vi "Insight_Telnet_VI_Test.vi"() -> ()   [LabVIEW 2011]
uses:
  Telnet Session.ctl
panel:
  out "Index of Synch Pulse":u32
  in  "Laser Write Values":T1={"Clock Rate (MHz)"=400.0, "num points"=0, "Duty Cycle (%)"=50.0, "Repetition Rate (kHz)"=200.0, "Start Wavelength (nm)"=1520.0, "Stop Wavelength (nm)"=1570.0, "Power (mW)"=1.0, "Power Profile"=enum."FLAT", "Sample Clock Delay (nsec)"=0.0, "Sweep Start Delay (nsec)"=0.0, "Data Valid Delay (nsec)"=0.0, "Optical Freq. Step (GHz)"=0.0, "Data Vector Length"=2000, "OPC Bit"=0}
  out "Invalid Data Indices":i32[](array[numeric])
  out "PLev Execution Timer (s)":dbl
  out "*IDN?":string
  out "Read Laser Settings":T1={"Clock Rate (MHz)"=400.0, "num points"=0, "Duty Cycle (%)"=50.0, "Repetition Rate (kHz)"=200.0, "Start Wavelength (nm)"=1520.0, "Stop Wavelength (nm)"=1570.0, "Power (mW)"=1.0, "Power Profile"=enum."FLAT", "Sample Clock Delay (nsec)"=0.0, "Sweep Start Delay (nsec)"=0.0, "Data Valid Delay (nsec)"=0.0, "Optical Freq. Step (GHz)"=0.0, "Data Vector Length"=2000, "OPC Bit"=0}
  in  "Mode":enum8{"Write", "Read"}(ring)=enum."Read"
  in  "Laser CMDs":T2(ring)
  in  "stop":bool
  out "error out":errorcluster
  in  "error in (no error)":errorcluster
  in  "IP Address":string="192.168.0.222"
  in  "Send Command":bool
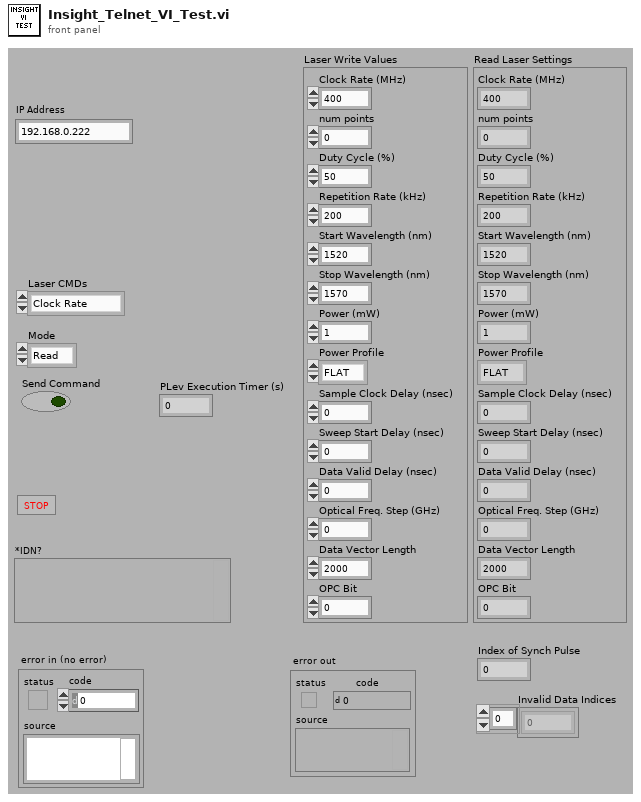
[diagram p1: front panel]
types:
  T1 = cluster{"Clock Rate (MHz)":dbl, "num points":u32, "Duty Cycle (%)":dbl, "Repetition Rate (kHz)":dbl, "Start Wavelength (nm)":dbl, "Stop Wavelength (nm)":dbl, "Power (mW)":dbl, "Power Profile":enum16{"FLAT", "GAUSsian"}, "Sample Clock Delay (nsec)":dbl, "Sweep Start Delay (nsec)":dbl, "Data Valid Delay (nsec)":dbl, "Optical Freq. Step (GHz)":dbl, "Data Vector Length":i32, "OPC Bit":u32}
  T2 = enum16{"Clock Rate", "Num Points", "Total Points", "Rep Rate", "DVV", "Freq Step", "StartWL", "StopWL", "Power", "Profile", "SCDelay", "SSDelay", "DVDelay", "Sync Index", "Synch Pulse", "Calibrate", "Abort", "Check OPC", "Get Parameters", "Power-Level", "Init Sweep"}
  T3 = typedef "Telnet Session.ctl" = refnum<k1>
  T4 = cluster{"Save Data Path":path, "Laser Serial Port":refnum<visa-resource-name>, "IP address":string, "remote port or service name":u16, "Laser connection ID":refnum<k5>, "telnet connection":T3, "*IDN":string, "OPC Bit":u32, "Counter":u32, "Measurement Complete?":bool, "Speed of Light (GHz-mm)":dbl, "Laser State":enum16{"Standby", "Calibrate", "Scan", "Fixed", "Idle"}, "Clock Rate (MHz)":dbl, "DAC Repeats":u32, "num points":u32, "Duty Cycle (%)":dbl, "Repetition Rate (kHz)":dbl, "Start Wavelength (nm)":dbl, "Stop Wavelength (nm)":dbl, "Power (mW)":dbl, "Power Profile":enum16{"FLAT", "GAUSsian"}, "Sample Clock Delay (nsec)":dbl, "Sweep Start Delay (nsec)":dbl, "Data Valid Delay (nsec)":dbl, "FFT Window":enum16{"Rectangular", "Hanning", "Hamming", "Blackman", "Blackman-Harris"}, "Data Vector Length":u32, "Optical Freq. Step (GHz)":dbl, "Distance Step (um)":dbl, "Indices of Data Invalid":i32[], "Raw Data":dbl[], "Data Valid":dbl[], "Processed Data":dbl[], "PSF":dbl[], "Distance Axis (mm)":dbl[], "Number of Measurements":i32, "PSF DataOut":cluster{"FW@3dB":dbl, "FW@20dB":dbl, "Ypeak":dbl, "Xpeak":dbl, "Dynamic \nRange":dbl, "WLRange (nm)":dbl}, "Program Message":string, "Data Acquisition Card":enum16{"Alazar Tech ATS9350", "SP Devices ADQ214"}, "adq_cu_ptr":u32, "adq214_num":i32, "Actual Laser Settings":cluster{"Clock Rate (MHz)":dbl, "num points":u32, "Duty Cycle (%)":dbl, "Repetition Rate (kHz)":dbl, "Start Wavelength (nm)":dbl, "Stop Wavelength (nm)":dbl, "Power (mW)":dbl, "Power Profile":enum16{"FLAT", "GAUSsian"}, "Sample Clock Delay (nsec)":dbl, "Sweep Start Delay (nsec)":dbl, "Data Valid Delay (nsec)":dbl, "Optical Freq. Step (GHz)":dbl, "Data Vector Length":i32, "OPC Bit":u32}, "Synch Data":dbl[][]}
  T5 = enum16{"Standby", "Calibrate", "Scan", "Fixed", "Idle"}
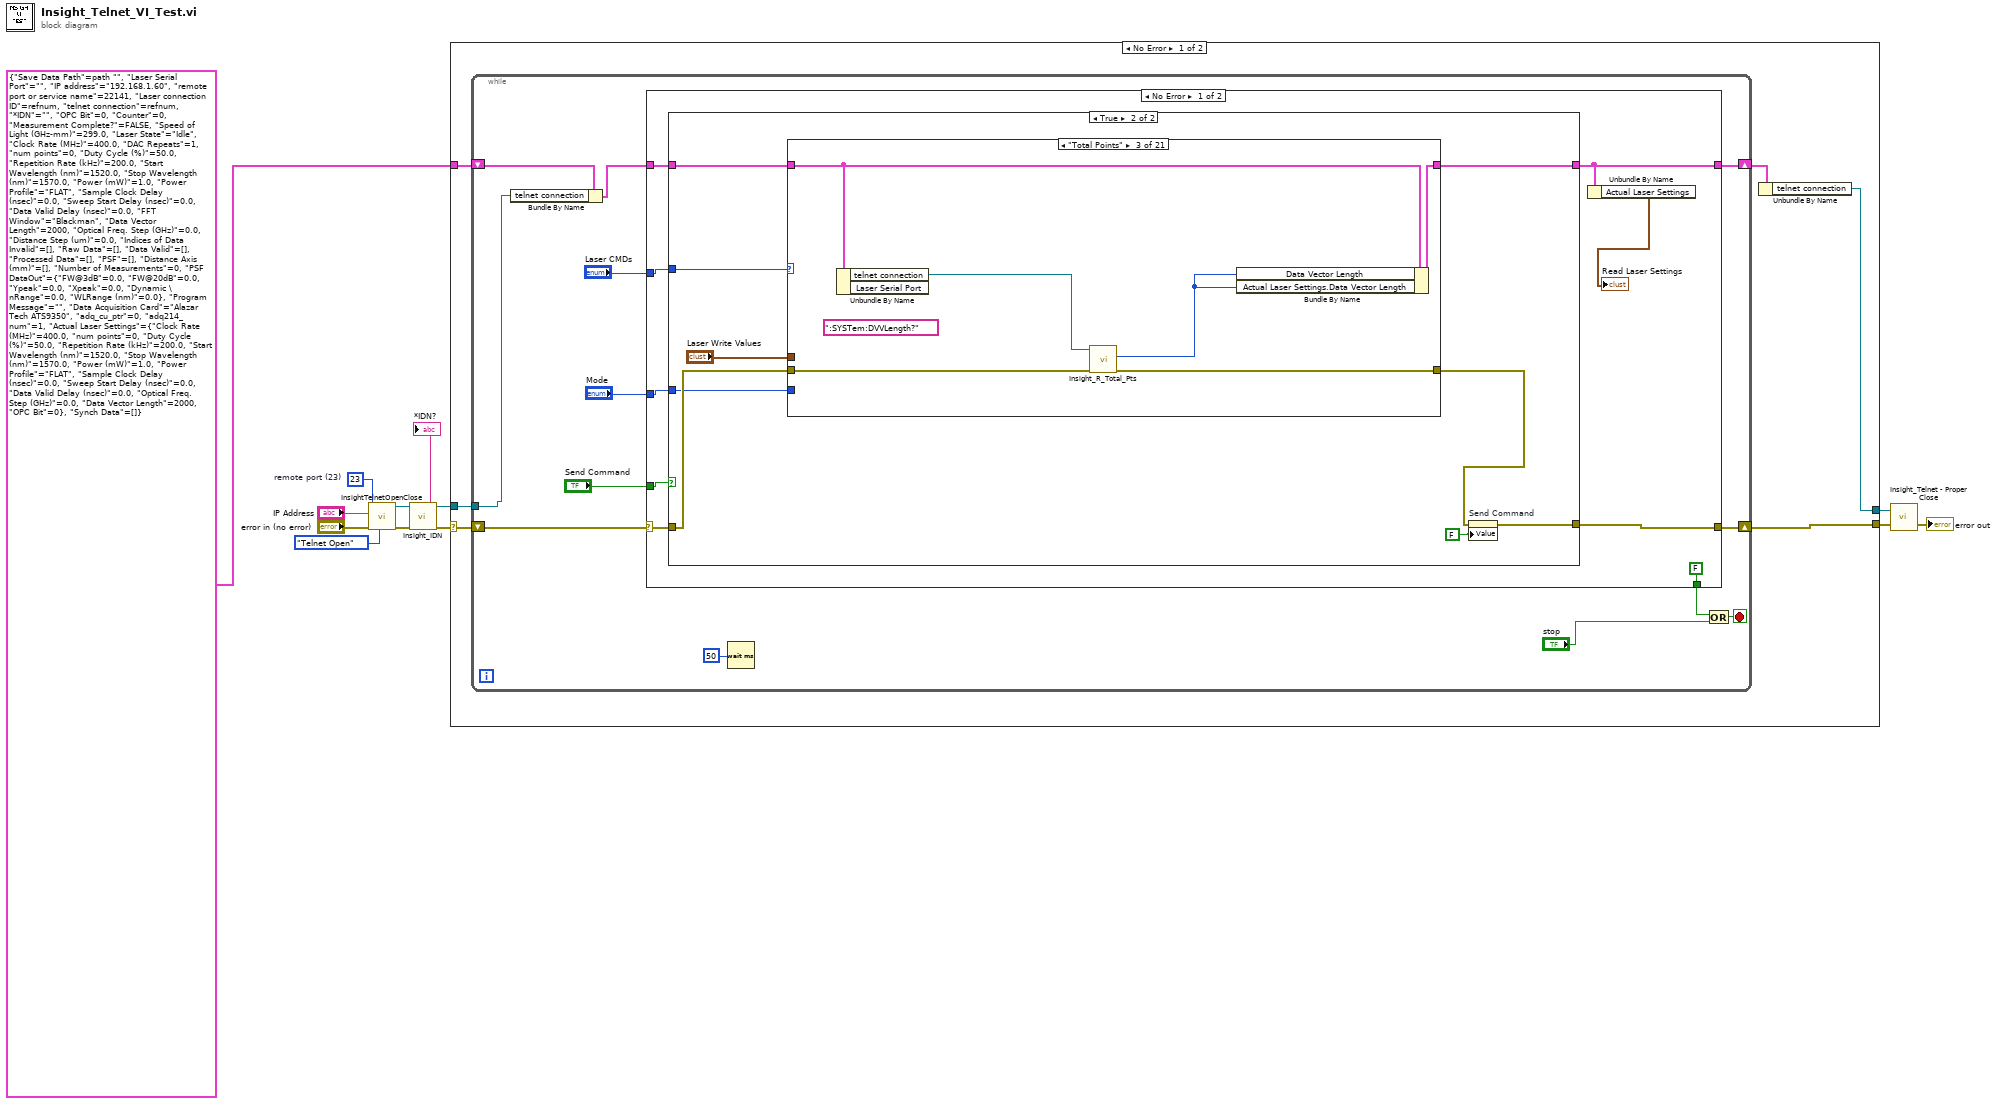
[diagram p0: block diagram]
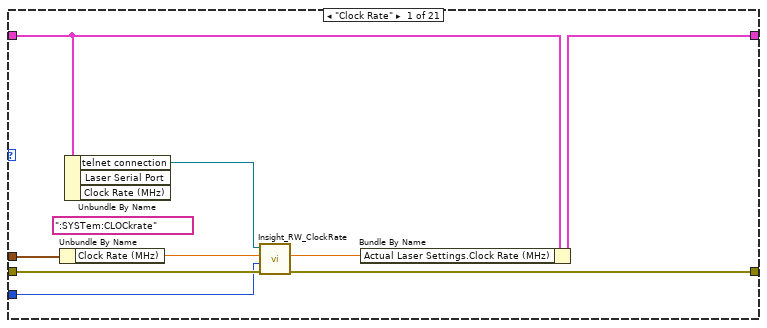
[diagram p3: hidden frame]
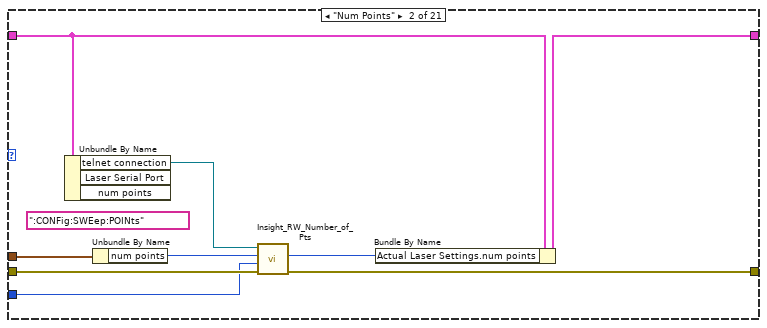
[diagram p4: hidden frame]
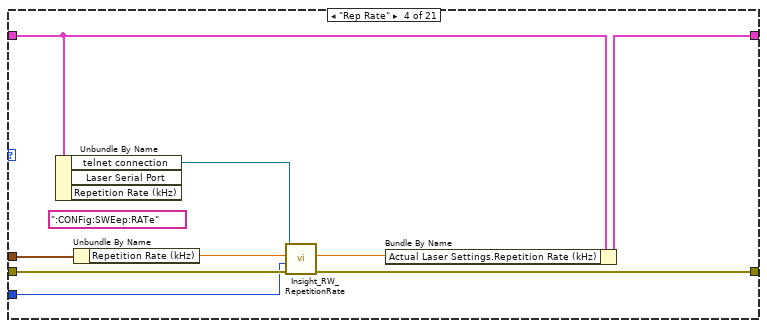
[diagram p5: hidden frame]
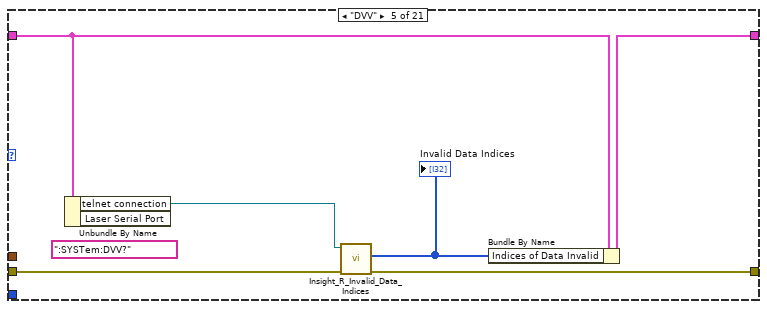
[diagram p6: hidden frame]
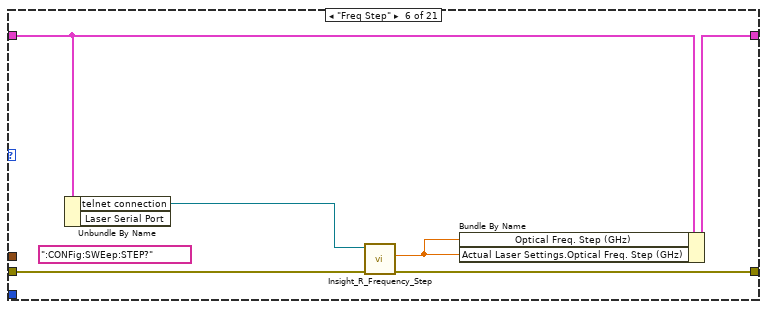
[diagram p7: hidden frame]
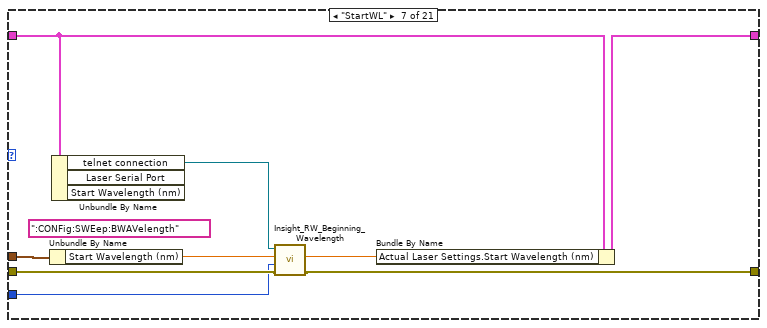
[diagram p8: hidden frame]
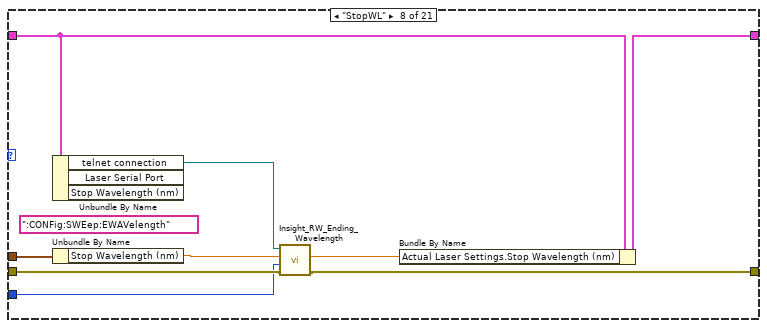
[diagram p9: hidden frame]
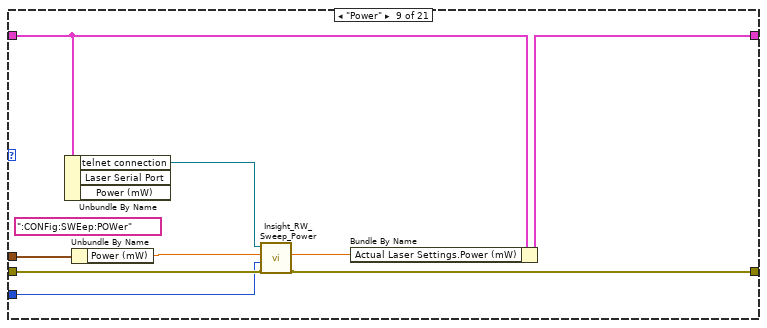
[diagram p10: hidden frame]
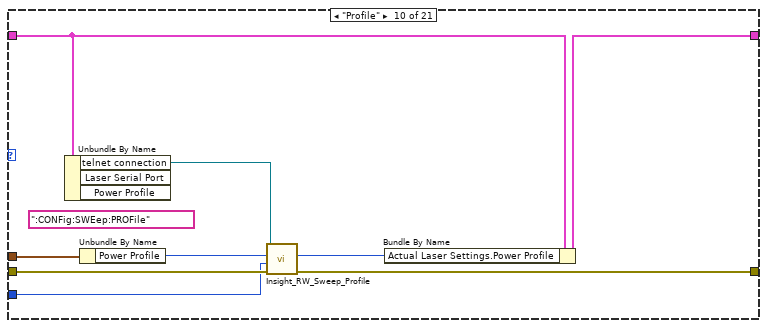
[diagram p11: hidden frame]
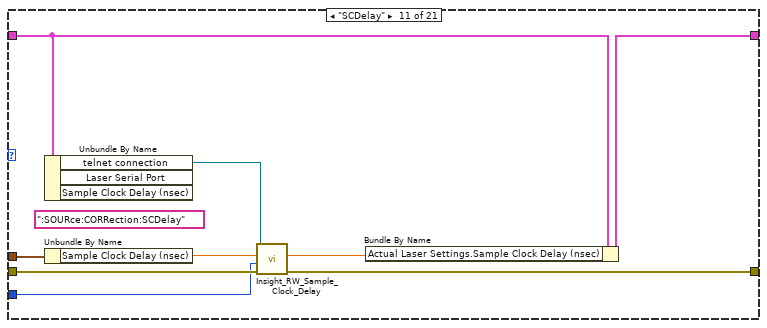
[diagram p12: hidden frame]
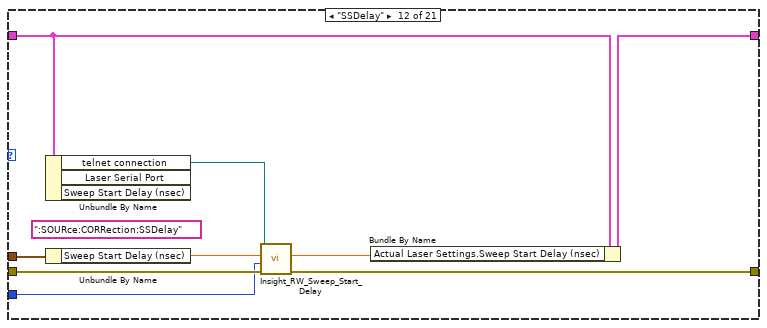
[diagram p13: hidden frame]
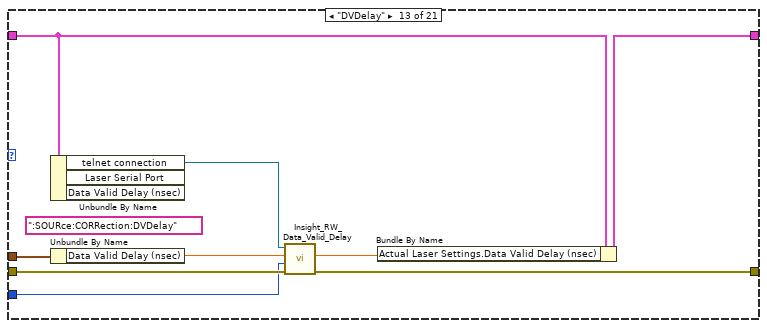
[diagram p14: hidden frame]
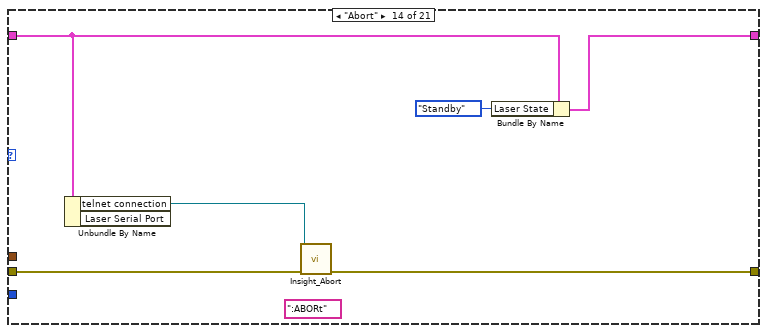
[diagram p15: hidden frame]
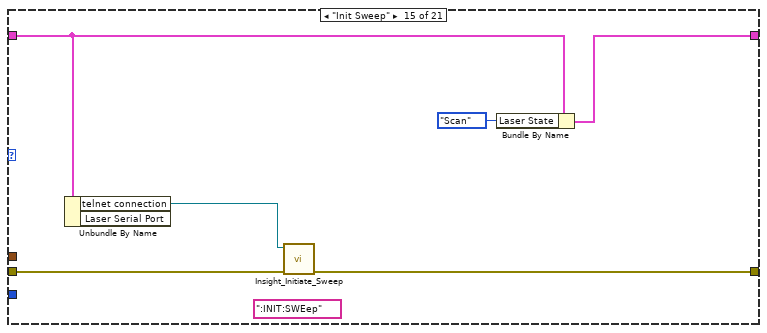
[diagram p16: hidden frame]
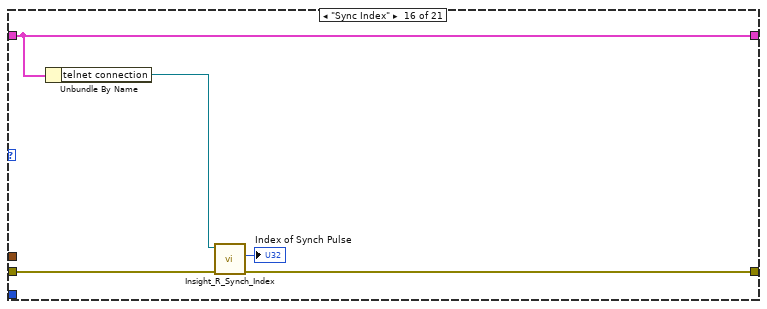
[diagram p17: hidden frame]
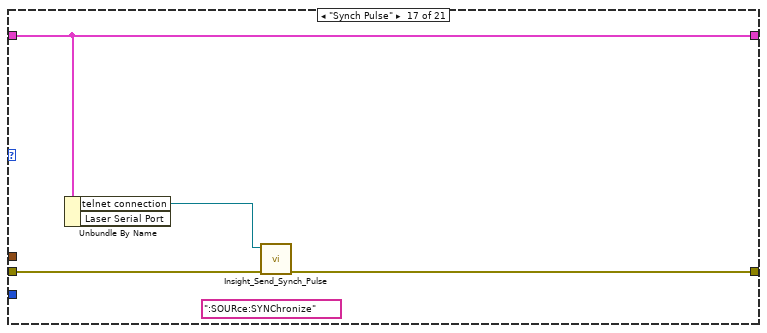
[diagram p18: hidden frame]
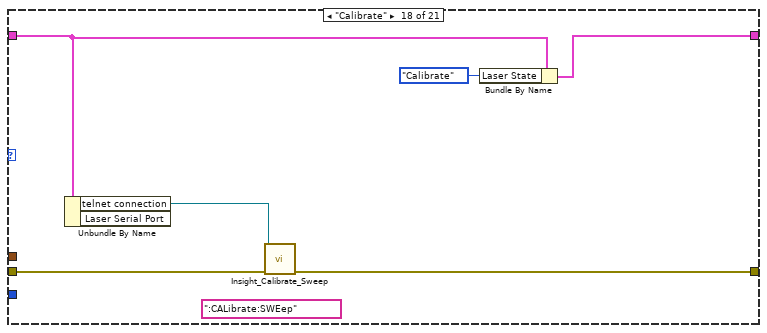
[diagram p19: hidden frame]
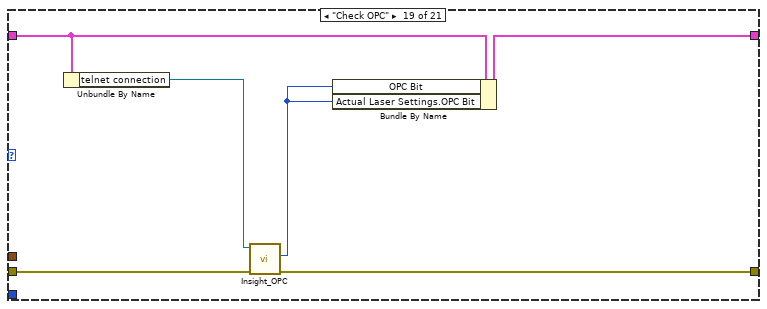
[diagram p20: hidden frame]
diagram:
  w1 = u16 23  # remote port (23)
  n1 = call "InsightTelnetOpenClose.vi"("IP Address"="IP Address", "remote port (23)"=w1, "error in (no error)"="error in (no error)", "Method"=enum16{"Telnet Open", "Telnet Close"}."Telnet Open") -> ("telnet connection"=w4:T3, "error out"=w6:errorcluster)  [unwired: 5 in]
  n2 = call "Insight_IDN.vi"("error in (no error)"=w6, "telnet connection"=w4) -> ("error out"=w5:errorcluster, "*IDN?"=→"*IDN?":string, "telnet  connection out"=w3:T3)  [unwired: 7 in]
  n3 = case shown="No Error" w5 {
    selector: w5 -> [w17 w220]
    tunnel: [w18 w220] -> w13
    tunnel: w3 -> [w19 w219]
    tunnel: [w14 w219] -> w12
    tunnel: T4 {"Save Data Path"=path "", "Laser Serial Port"="", "IP address"="192.168.1.60", "remote port or service name"=22141, "Laser connection ID"=refnum, "telnet connection"=refnum, "*IDN"="", "OPC Bit"=0, "Counter"=0, "Measurement Complete?"=FALSE, "Speed of Light (GHz-mm)"=299.0, "Laser State"=enum."Idle", "Clock Rate (MHz)"=400.0, "DAC Repeats"=1, "num points"=0, "Duty Cycle (%)"=50.0, "Repetition Rate (kHz)"=200.0, "Start Wavelength (nm)"=1520.0, "Stop Wavelength (nm)"=1570.0, "Power (mW)"=1.0, "Power Profile"=enum."FLAT", "Sample Clock Delay (nsec)"=0.0, "Sweep Start Delay (nsec)"=0.0, "Data Valid Delay (nsec)"=0.0, "FFT Window"=enum."Blackman", "Data Vector Length"=2000, "Optical Freq. Step (GHz)"=0.0, "Distance Step (um)"=0.0, "Indices of Data Invalid"=[], "Raw Data"=[], "Data Valid"=[], "Processed Data"=[], "PSF"=[], "Distance Axis (mm)"=[], "Number of Measurements"=0, "PSF DataOut"={"FW@3dB"=0.0, "FW@20dB"=0.0, "Ypeak"=0.0, "Xpeak"=0.0, "Dynamic \nRange"=0.0, "WLRange (nm)"=0.0}, "Program Message"="", "Data Acquisition Card"=enum."Alazar Tech ATS9350", "adq_cu_ptr"=0, "adq214_num"=1, "Actual Laser Settings"={"Clock Rate (MHz)"=400.0, "num points"=0, "Duty Cycle (%)"=50.0, "Repetition Rate (kHz)"=200.0, "Start Wavelength (nm)"=1520.0, "Stop Wavelength (nm)"=1570.0, "Power (mW)"=1.0, "Power Profile"=enum."FLAT", "Sample Clock Delay (nsec)"=0.0, "Sweep Start Delay (nsec)"=0.0, "Data Valid Delay (nsec)"=0.0, "Optical Freq. Step (GHz)"=0.0, "Data Vector Length"=2000, "OPC Bit"=0}, "Synch Data"=[]} -> [w16 _]
    frame No Error {
      n4 = while {
        tunnel: w19 -> [w20]
        shift-right: [w30] -> w18
        shift-left: w17 -> [w29]
        shift-right: [w25] -> w15
        shift-left: w16 -> [w22]
        stop <- w26 stop-if-true
        n5 = Bundle By Name(cluster=w22, "telnet connection"=w20) -> (w21:T4)
        n6 = case shown="No Error" w29 {
          selector: w29 -> [w39 w218]
          tunnel: "Send Command" -> [w41 _]
          tunnel: [w40 w218] -> w30
          tunnel: [FALSE TRUE] -> w28
          tunnel: w21 -> [w37 w216]
          tunnel: [w34 w216] -> w25
          tunnel: "Laser CMDs" -> [w36 _]
          tunnel: "Mode" -> [w35 _]
          frame No Error {
            n7 = case shown="True" w41 {
              tunnel: w39 -> [w43 w47]
              tunnel: [w43 w51] -> w40
              tunnel: w37 -> [w42 w49]
              tunnel: [w42 w48] -> w34
              tunnel: w36 -> [_ w46]
              tunnel: w35 -> [_ w45]
              frame False {
              }
              frame True {
                n8 = case shown="\"Total Points\"" w46 {
                  tunnel: w49 -> [w61 w70 w76 w85 w91 w97 w106 w115 w124 w133 w142 w151 w160 w166 w172 w177 w181 w186 w190 w195 w197]
                  tunnel: w47 -> [w59 w68 w74 w83 w89 w95 w104 w113 w122 w131 w140 w149 w158 w162 w169 w176 w179 w184 w193 w194 w203]
                  tunnel: [w60 w69 w75 w84 w90 w96 w105 w114 w123 w132 w141 w150 w159 w165 w171 w177 w181 w185 w189 w195 w197] -> w48
                  tunnel: [w58 w67 w73 w82 w88 w94 w103 w112 w121 w130 w139 w148 w157 w161 w168 w174 w180 w183 w192 w194 w198] -> w50
                  tunnel: w45 -> [w55 w64 _ w79 _ _ w101 w110 w118 w129 w136 w145 w154 _ _ _ _ _ _ _ _]
                  tunnel: "Laser Write Values" -> [w54 w63 _ w77 _ _ w99 w108 w117 w126 w135 w144 w153 _ _ _ _ _ _ _ _]
                  frame "Clock Rate" {
                    (unwired) ":SYSTem:CLOCkrate" ("String")
                    n9 = Unbundle By Name(w54) -> ("Clock Rate (MHz)"=w53:dbl)
                    n10 = Unbundle By Name(w61) -> ("telnet connection"=w56:T3)  [unwired: 2 out]
                    n11 = call "Insight_RW_ClockRate.vi"("error in (no error)"=w59, "Mode (Read / Write)"=w55, "Clock Rate (MHz)"=w53, "telnet connection"=w56) -> ("error out"=w58:errorcluster, "Clock Rate (MHz)"=w57:dbl)  [unwired: 4 in, 2 out]
                    n12 = Bundle By Name(cluster=w61, "Actual Laser Settings.Clock Rate (MHz)"=w57) -> (w60:T4)
                  }
                  frame "Num Points" {
                    (unwired) ":CONFig:SWEep:POINts" ("String")
                    n13 = Unbundle By Name(w70) -> ("telnet connection"=w65:T3)  [unwired: 2 out]
                    n14 = Unbundle By Name(w63) -> ("num points"=w62:u32)
                    n15 = call "Insight_RW_Number_of_Pts.vi"("error in (no error)"=w68, "Mode (Read / Write)"=w64, "Number of Points"=w62, "telnet connection"=w65) -> ("error out"=w67:errorcluster, "Number of Points"=w66:u32)  [unwired: 4 in, 2 out]
                    n16 = Bundle By Name(cluster=w70, "Actual Laser Settings.num points"=w66) -> (w69:T4)
                  }
                  frame "Total Points" {
                    (unwired) ":SYSTem:DVVLength?" ("String")
                    n17 = Unbundle By Name(w76) -> ("telnet connection"=w71:T3)  [unwired: 1 out]
                    n18 = call "Insight_R_Total_Pts.vi"("error in (no error)"=w74, "telnet connection"=w71) -> ("error out"=w73:errorcluster, "Total Points"=w72:u32)  [unwired: 6 in, 2 out]
                    n19 = Bundle By Name(cluster=w76, "Data Vector Length"=w72, "Actual Laser Settings.Data Vector Length"=w72) -> (w75:T4)
                  }
                  frame "Rep Rate" {
                    (unwired) ":CONFig:SWEep:RATe" ("String")
                    n20 = Unbundle By Name(w85) -> ("telnet connection"=w80:T3)  [unwired: 2 out]
                    n21 = Unbundle By Name(w77) -> ("Repetition Rate (kHz)"=w78:dbl)
                    n22 = call "Insight_RW_RepetitionRate.vi"("error in (no error)"=w83, "Mode (Read / Write)"=w79, "Repetition Rate (kHz)"=w78, "telnet connection"=w80) -> ("error out"=w82:errorcluster, "Repetition Rate (kHz)"=w81:dbl)  [unwired: 4 in, 2 out]
                    n23 = Bundle By Name(cluster=w85, "Actual Laser Settings.Repetition Rate (kHz)"=w81) -> (w84:T4)
                  }
                  frame "DVV" {
                    (unwired) ":SYSTem:DVV?" ("String")
                    n24 = Unbundle By Name(w91) -> ("telnet connection"=w87:T3)  [unwired: 1 out]
                    n25 = call "Insight_R_Invalid_Data_Indices.vi"("error in (no error)"=w89, "telnet connection"=w87) -> ("error out"=w88:errorcluster, "Invalid Data Indices"=w86:i32[])  [unwired: 6 in, 2 out]
                    "Invalid Data Indices" <- w86
                    n26 = Bundle By Name(cluster=w91, "Indices of Data Invalid"=w86) -> (w90:T4)
                  }
                  frame "Freq Step" {
                    (unwired) ":CONFig:SWEep:STEP?" ("String")
                    n27 = Unbundle By Name(w97) -> ("telnet connection"=w93:T3)  [unwired: 1 out]
                    n28 = call "Insight_R_Frequency_Step.vi"("error in (no error)"=w95, "telnet connection"=w93) -> ("error out"=w94:errorcluster, "Optical Frequency Step (GHz)"=w92:dbl)  [unwired: 6 in, 2 out]
                    n29 = Bundle By Name(cluster=w97, "Optical Freq. Step (GHz)"=w92, "Actual Laser Settings.Optical Freq. Step (GHz)"=w92) -> (w96:T4)
                  }
                  frame "StartWL" {
                    (unwired) ":CONFig:SWEep:BWAVelength" ("String")
                    n30 = Unbundle By Name(w99) -> ("Start Wavelength (nm)"=w98:dbl)
                    n31 = Unbundle By Name(w106) -> ("telnet connection"=w102:T3)  [unwired: 2 out]
                    n32 = call "Insight_RW_Beginning_Wavelength.vi"("error in (no error)"=w104, "Mode (Read / Write)"=w101, "Beginning Wavelength (nm)"=w98, "telnet connection"=w102) -> ("error out"=w103:errorcluster, "Beginning Wavelength (nm)"=w100:dbl)  [unwired: 4 in, 2 out]
                    n33 = Bundle By Name(cluster=w106, "Actual Laser Settings.Start Wavelength (nm)"=w100) -> (w105:T4)
                  }
                  frame "StopWL" {
                    (unwired) ":CONFig:SWEep:EWAVelength" ("String")
                    n34 = Unbundle By Name(w115) -> ("telnet connection"=w111:T3)  [unwired: 2 out]
                    n35 = Unbundle By Name(w108) -> ("Stop Wavelength (nm)"=w107:dbl)
                    n36 = call "Insight_RW_Ending_Wavelength.vi"("error in (no error)"=w113, "Mode (Read / Write)"=w110, "Ending Wavelength (nm)"=w107, "telnet connection"=w111) -> ("error out"=w112:errorcluster, "Ending Wavelength (nm)"=w109:dbl)  [unwired: 4 in, 2 out]
                    n37 = Bundle By Name(cluster=w115, "Actual Laser Settings.Stop Wavelength (nm)"=w109) -> (w114:T4)
                  }
                  frame "Power" {
                    (unwired) ":CONFig:SWEep:POWer" ("String")
                    n38 = Unbundle By Name(w124) -> ("telnet connection"=w119:T3)  [unwired: 2 out]
                    n39 = Unbundle By Name(w117) -> ("Power (mW)"=w116:dbl)
                    n40 = call "Insight_RW_Sweep_Power.vi"("error in (no error)"=w122, "Mode (Read / Write)"=w118, "Power (mW)"=w116, "telnet connection"=w119) -> ("error out"=w121:errorcluster, "Power (mW)"=w120:dbl)  [unwired: 4 in, 2 out]
                    n41 = Bundle By Name(cluster=w124, "Actual Laser Settings.Power (mW)"=w120) -> (w123:T4)
                  }
                  frame "Profile" {
                    (unwired) ":CONFig:SWEep:PROFile" ("String")
                    n42 = Unbundle By Name(w133) -> ("telnet connection"=w128:T3)  [unwired: 2 out]
                    n43 = Unbundle By Name(w126) -> ("Power Profile"=w125:enum16{"FLAT", "GAUSsian"})
                    n44 = call "Insight_RW_Sweep_Profile.vi"("error in (no error)"=w131, "Mode (Read / Write)"=w129, "Power Profile"=w125, "telnet connection"=w128) -> ("error out"=w130:errorcluster, "Power Profile"=w127:enum16{"FLAT", "GAUSsian"})  [unwired: 4 in, 2 out]
                    n45 = Bundle By Name(cluster=w133, "Actual Laser Settings.Power Profile"=w127) -> (w132:T4)
                  }
                  frame "SCDelay" {
                    (unwired) ":SOURce:CORRection:SCDelay" ("String")
                    n46 = Unbundle By Name(w142) -> ("telnet connection"=w138:T3)  [unwired: 2 out]
                    n47 = Unbundle By Name(w135) -> ("Sample Clock Delay (nsec)"=w134:dbl)
                    n48 = call "Insight_RW_Sample_Clock_Delay.vi"("error in (no error)"=w140, "Mode (Read / Write)"=w136, "Sample Clock Delay (nsec)"=w134, "telnet connection"=w138) -> ("error out"=w139:errorcluster, "Sample Clock Delay (nsec)"=w137:dbl)  [unwired: 4 in, 2 out]
                    n49 = Bundle By Name(cluster=w142, "Actual Laser Settings.Sample Clock Delay (nsec)"=w137) -> (w141:T4)
                  }
                  frame "SSDelay" {
                    (unwired) ":SOURce:CORRection:SSDelay" ("String")
                    n50 = Unbundle By Name(w151) -> ("telnet connection"=w146:T3)  [unwired: 2 out]
                    n51 = Unbundle By Name(w144) -> ("Sweep Start Delay (nsec)"=w143:dbl)
                    n52 = call "Insight_RW_Sweep_Start_Delay.vi"("error in (no error)"=w149, "Mode (Read / Write)"=w145, "Sweep Start Delay (nsec)"=w143, "telnet connection"=w146) -> ("error out"=w148:errorcluster, "Sweep Start Delay (nsec)"=w147:dbl)  [unwired: 4 in, 2 out]
                    n53 = Bundle By Name(cluster=w151, "Actual Laser Settings.Sweep Start Delay (nsec)"=w147) -> (w150:T4)
                  }
                  frame "DVDelay" {
                    (unwired) ":SOURce:CORRection:DVDelay" ("String")
                    n54 = Unbundle By Name(w160) -> ("telnet connection"=w155:T3)  [unwired: 2 out]
                    n55 = Unbundle By Name(w153) -> ("Data Valid Delay (nsec)"=w152:dbl)
                    n56 = call "Insight_RW_Data_Valid_Delay.vi"("error in (no error)"=w158, "Mode (Read / Write)"=w154, "Data Valid Delay (nsec)"=w152, "telnet connection"=w155) -> ("error out"=w157:errorcluster, "Data Valid Delay (nsec)"=w156:dbl)  [unwired: 4 in, 2 out]
                    n57 = Bundle By Name(cluster=w160, "Actual Laser Settings.Data Valid Delay (nsec)"=w156) -> (w159:T4)
                  }
                  frame "Abort" {
                    (unwired) ":ABORt" ("String")
                    n58 = Unbundle By Name(w166) -> ("telnet connection"=w163:T3)  [unwired: 1 out]
                    n59 = call "Insight_Abort.vi"("error in (no error)"=w162, "telnet connection"=w163) -> ("error out"=w161:errorcluster)  [unwired: 7 in, 2 out]
                    n60 = Bundle By Name(cluster=w166, "Laser State"=T5."Standby") -> (w165:T4)
                  }
                  frame "Init Sweep" {
                    (unwired) ":INIT:SWEep" ("String")
                    n61 = Unbundle By Name(w172) -> ("telnet connection"=w167:T3)  [unwired: 1 out]
                    n62 = call "Insight_Initiate_Sweep.vi"("error in (no error)"=w169, "telnet connection"=w167) -> ("error out"=w168:errorcluster)  [unwired: 7 in, 2 out]
                    n63 = Bundle By Name(cluster=w172, "Laser State"=T5."Scan") -> (w171:T4)
                  }
                  frame "Sync Index" {
                    n64 = Unbundle By Name(w177) -> ("telnet connection"=w175:T3)
                    n65 = call "Insight_R_Synch_Index.vi"("error in (no error)"=w176, "telnet connection"=w175) -> ("error out"=w174:errorcluster, "Index of Synch Pulse"=→"Index of Synch Pulse":u32)  [unwired: 6 in, 2 out]
                  }
                  frame "Synch Pulse" {
                    (unwired) ":SOURce:SYNChronize" ("String")
                    n66 = Unbundle By Name(w181) -> ("telnet connection"=w178:T3)  [unwired: 1 out]
                    n67 = call "Insight_Send_Synch_Pulse.vi"("error in (no error)"=w179, "telnet connection"=w178) -> ("error out"=w180:errorcluster)  [unwired: 7 in, 2 out]
                  }
                  frame "Calibrate" {
                    (unwired) ":CALibrate:SWEep" ("String")
                    n68 = Unbundle By Name(w186) -> ("telnet connection"=w182:T3)  [unwired: 1 out]
                    n69 = call "Insight_Calibrate_Sweep.vi"("error in (no error)"=w184, "telnet connection"=w182) -> ("error out"=w183:errorcluster)  [unwired: 7 in, 2 out]
                    n70 = Bundle By Name(cluster=w186, "Laser State"=T5."Calibrate") -> (w185:T4)
                  }
                  frame "Check OPC" {
                    n71 = Unbundle By Name(w190) -> ("telnet connection"=w191:T3)
                    n72 = call "Insight_OPC.vi"("error in (no error)"=w193, "telnet connection"=w191) -> ("error out"=w192:errorcluster, "OPC Bit value (1=Idle)"=w188:u32)  [unwired: 6 in, 2 out]
                    n73 = Bundle By Name(cluster=w190, "OPC Bit"=w188, "Actual Laser Settings.OPC Bit"=w188) -> (w189:T4)
                  }
                  frame "Get Parameters" {
                    (unwired) string[] ["CMD Clock Rate?", "CMD Num Points?", "CMD Total Points?", "CMD Rep Rate?", "CMD Freq Step?", "CMD StartWL?", "CMD StopWL?", "CMD Power?", "CMD Profile?", "CMD SCDelay?", "CMD SSDelay?", "CMD DVDelay?", "update display"] ("queue array")
                    # "Install all parameter reads"
                  }
                  frame "Power-Level" {
                    n74 = Unbundle By Name(w197) -> ("telnet connection"=w202:T3)
                    n75 = call "InsightTelnetComm.vi"("error in"=w203, "Timeout, sec"=u32 3, "write buffer (\"\")"=":diag:utest:plev" ("write buffer (\"\")"), "telnet connection"=w202) -> ("error out"=w200:errorcluster, "telnet  connection out"=w199:T3)  [unwired: 3 in, 1 out]
                    n76 = while {
                      tunnel: w200 -> [w213]
                      tunnel: w199 -> [w210]
                      tunnel: [w209] -> w198
                      i -> [w207]
                      stop <- w208 stop-if-true
                      n77 = flat-sequence {
                        tunnel: w213 -> [w215]
                        tunnel: [w215] -> w212
                        tunnel: [w214] -> w206
                        frame #0 {
                          w214 = u32 1000 ("milliseconds to wait")
                          n78 = Wait (ms)(milliseconds to wait=w214) -> ()  [unwired: 1 out]
                        }
                      }
                      n79 = Compound Arithmetic op=MULTIPLY(w207, w206, 0.001 ("value")) -> (→"PLev Execution Timer (s)":dbl)
                      n80 = call "Insight_OPC.vi"("error in (no error)"=w212, "telnet connection"=w210) -> ("error out"=w209:errorcluster, "OPC Bit value (1=Idle)"=w211:u32)  [unwired: 6 in, 2 out]
                      n81 = Not Equal To 0?(x=w211) -> (x != 0?=w208:bool)
                    }
                  }
                }
                n82 = property on="Send Command" class="Bool (strict)"(error in=w50, "Value"=FALSE ("Send Command")) -> (error out=w51:errorcluster)  [unwired: 1 in, 1 out]
              }
            }
            n83 = Unbundle By Name(w34) -> ("Actual Laser Settings"=→"Read Laser Settings":T1)
          }
          frame Error {
          }
        }
        n84 = Wait (ms)(milliseconds to wait=u32 50) -> ()  [unwired: 1 out]
        n85 = Or(x=w28, y="stop") -> (x .or. y?=w26:bool)
      }
      n86 = Unbundle By Name(w15) -> ("telnet connection"=w14:T3)
    }
    frame Error {
    }
  }
  n87 = call "Insight_Telnet - Proper Close.vi"("error in"=w13, "telnet connection"=w12) -> ("error out"=→"error out":errorcluster)  [unwired: 1 in]
